vi "Drag Control Point.vi"(0 "FSM.Edge In":refnum<class "FSM.Edge.lvclass">, 9 "location":T1) -> (4 "FSM.Edge Out":refnum<class "FSM.Edge.lvclass">)   [LabVIEW 2020, in "FSM.Edge.lvclass"]
uses:
  FSM.Edge.lvclass
  <vilib>/Utility/miscctls.llb/LVPoint32TypeDef.ctl
  FSM.Edge.lvclass/FSM.Edge.ctl
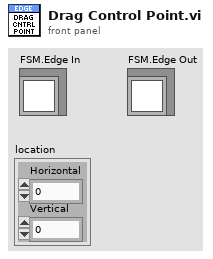
[diagram p1: front panel]
types:
  T1 = typedef "LVPoint32TypeDef.ctl" = cluster{"Horizontal":i32, "Vertical":i32}
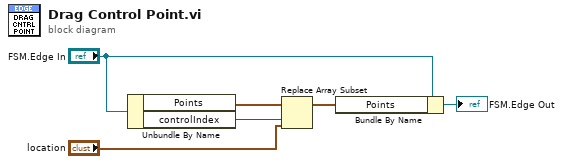
[diagram p0: block diagram]
diagram:
  n1 = Unbundle By Name("FSM.Edge In") -> ("Points"=w4:cluster{"x":i16, "y":i16}[], "controlIndex"=w3:i32)
  n2 = Replace Array Subset(array=w4, new element="location", index=w3) -> (w1:cluster{"x":i16, "y":i16}[])
  n3 = Bundle By Name(cluster="FSM.Edge In", "Points"=w1) -> (→"FSM.Edge Out":refnum<class "FSM.Edge.lvclass">)
